vi "Intake Jam.vi"(9 "Power":dbl, 10 "Surge":dbl, 11 "MotorControlDevRef":T1) -> (3 "Front Jam":bool)   [LabVIEW 2019]
uses:
  <vilib>/Rock Robotics/WPI/MotorControl/WPI_MotorControlDeviceRef.ctl
  <vilib>/Rock Robotics/WPI/MotorControl/WPI_MotorControlType.ctl
  <vilib>/Rock Robotics/SystemInterfaces/DIO/FPGA_DIOPWMChannel.ctl
  <vilib>/Rock Robotics/WPI/PWM/WPI_PWMDeadband.ctl
  <vilib>/Rock Robotics/SystemInterfaces/DIO/FPGA_DIOChannel.ctl
  <vilib>/ptbypt/NI_PtbyPt.lvlib
panel:
  in  "dt":u32
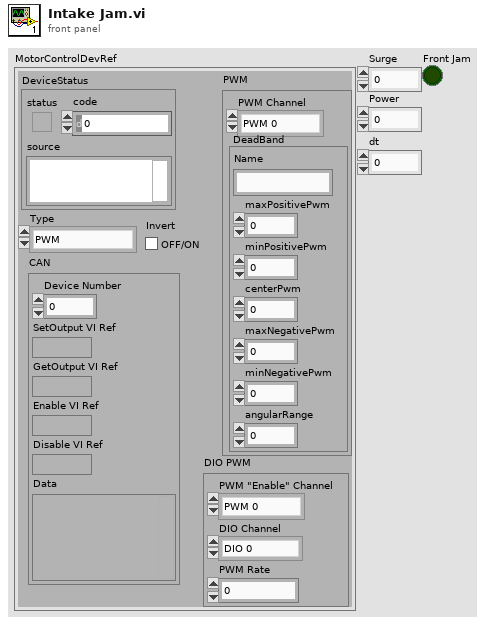
[diagram p1: front panel]
types:
  T1 = typedef "WPI_MotorControlDeviceRef.ctl" = cluster{"DeviceStatus":errorcluster, "Type":T2, "PWM":cluster{"PWM Channel":T3, "DeadBand":T4}, "CAN":cluster{"Device Number":u8, "SetOutput VI Ref":variant, "GetOutput VI Ref":variant, "Enable VI Ref":variant, "Disable VI Ref":variant, "Data":variant}, "Invert":bool, "DIO PWM":cluster{"PWM \"Enable\" Channel":T3, "DIOChannel":T5, "PWM Rate":dbl}}
  T2 = typedef "WPI_MotorControlType.ctl" = enum16{"PWM", "CAN", "DIO PWM"}
  T3 = typedef "FPGA_DIOPWMChannel.ctl" = enum8{"PWM 0", "PWM 1", "PWM 2", "PWM 3", "PWM 4", "PWM 5", "PWM 6", "PWM 7", "PWM 8", "PWM 9", "PWM MXP 0", "PWM MXP 1", "PWM MXP 2", "PWM MXP 3", "PWM MXP 4", "PWM MXP 5", "PWM MXP 6", "PWM MXP 7", "PWM MXP 8", "PWM MXP 9", "Invalid"}
  T4 = typedef "WPI_PWMDeadband.ctl" = cluster{"Name":string, "maxPositivePwm":i32, "minPositivePwm":i32, "centerPwm":i32, "maxNegativePwm":i32, "minNegativePwm":i32, "angularRange":u16}
  T5 = typedef "FPGA_DIOChannel.ctl" = enum8{"DIO 0", "DIO 1", "DIO 2", "DIO 3", "DIO 4", "DIO 5", "DIO 6", "DIO 7", "DIO 8", "DIO 9", "DIO MXP 0", "DIO MXP 1", "DIO MXP 2", "DIO MXP 3", "DIO MXP 4", "DIO MXP 5", "DIO MXP 6", "DIO MXP 7", "DIO MXP 8", "DIO MXP 9", "DIO MXP 10", "DIO MXP 11", "DIO MXP 12", "DIO MXP 13", "DIO MXP 14", "DIO MXP 15", "SPI Port CS1", "SPI Port CS2", "SPI Port CS3", "SPI Port MISO", "SPI Port MOSI", "Invalid"}
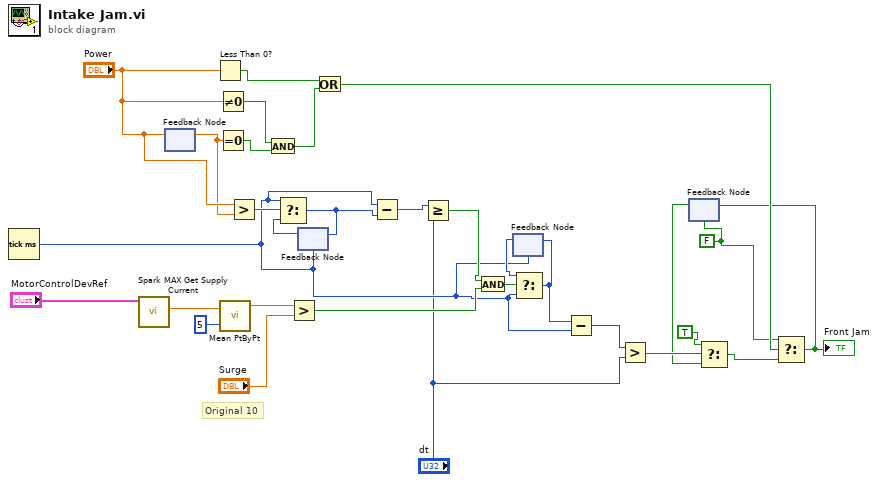
[diagram p0: block diagram]
diagram:
  w9 = FALSE
  # "Original 10"
  n1 = Tick Count (ms)() -> (millisecond timer value=w15:u32)
  n2 = call <vilib>:"Spark MAX Get Supply Current.vi"("MotorControlDevRef in"="MotorControlDevRef") -> ("Current"=w29:dbl)  [unwired: 7 in, 3 out]
  n3 = feedback-in #1("Power") -> ()
  n4 = feedback #1() -> (w3:dbl)  [unwired: 1 in]
  n5 = Less Than 0?(x="Power") -> (x < 0?=w25:bool)
  n6 = Not Equal To 0?(x="Power") -> (x != 0?=w5:bool)
  n7 = Equal To 0?(x=w3) -> (x = 0?=w4:bool)
  n8 = call <vilib>:"Mean PtByPt.vi"("x"=w29, "sample length"=5) -> ("mean"=w27:dbl)  [unwired: 2 in, 1 out]
  n9 = Greater?(x="Power", y=w3) -> (0:w23:bool)
  n10 = And(x=w5, y=w4) -> (x .and. y?=w24:bool)
  n11 = Greater?(x=w27, y="Surge") -> (0:w19:bool)
  n12 = feedback #2(w15) -> (w22:u32)
  n13 = Select(t=w15, s=w23, f=w22) -> (s? t:f=w21:u32)
  n14 = feedback-in #2(w21) -> ()
  n15 = Or(x=w25, y=w24) -> (x .or. y?=w10:bool)
  n16 = Subtract(x=w15, y=w21) -> (x-y=w2:u32)
  n17 = Greater Or Equal?(x=w2, y="dt") -> (x >= y?=w20:bool)
  n18 = And(x=w20, y=w19) -> (x .and. y?=w18:bool)
  n19 = feedback #3(w15) -> (w17:u32)
  n20 = Select(t=w17, s=w18, f=w15) -> (s? t:f=w16:u32)
  n21 = feedback-in #3(w16) -> ()
  n22 = Subtract(x=w16, y=w15) -> (x-y=w14:u32)
  n23 = Greater?(x=w14, y="dt") -> (0:w13:bool)
  n24 = feedback #4(w9) -> (w11:bool)
  n25 = Select(t=TRUE, s=w13, f=w11) -> (s? t:f=w8:bool)
  n26 = Select(t=w9, s=w10, f=w8) -> (s? t:f=w7:bool)
  "Front Jam" <- w7
  n27 = feedback-in #4(w7) -> ()
